vi "Events.vi"(8 "error in (no error)":errorcluster, 11 "LocalEventCollector in":refnum<class "LocalEventCollector.lvclass">) -> (0 "error out":errorcluster, 2 "Events":T1[](array[typedef]), 3 "LocalEventCollector out":refnum<class "LocalEventCollector.lvclass">)   [LabVIEW 2020, in "Vecto.lvlib" / "LocalEventCollector.lvclass"]
uses:
  LocalEventCollector.lvclass
  Event.ctl
  lv-volatus/Volatus/Event Level.ctl
  LocalEventCollector.lvclass/LocalEventCollector.ctl
  lv-volatus/Volatus/Volatus.lvlib
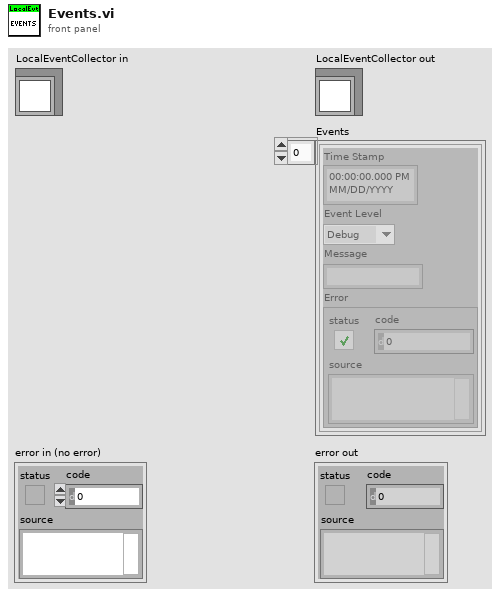
[diagram p1: front panel]
types:
  T1 = typedef "Vecto.lvlib/LocalEventCollector.lvclass/Event.ctl" = cluster{"Time Stamp":timestamp, "Event Level":T2, "Message":string, "Error":errorcluster}
  T2 = typedef "Volatus.lvlib/Event Level.ctl" = enum16{"Debug", "Info", "Warning", "Error"}
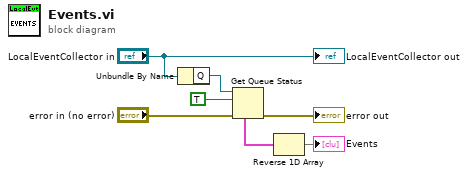
[diagram p0: block diagram]
diagram:
  n1 = Unbundle By Name("LocalEventCollector in") -> ("Q"=w6:refnum<queue>)
  n2 = Get Queue Status(queue=w6, return elements? (F)=TRUE, error in (no error)="error in (no error)") -> (error out=→"error out":errorcluster, elements=w4:T1[])  [unwired: 6 out]
  n3 = Reverse 1D Array(array=w4) -> (reversed array=→"Events":T1[])
  "LocalEventCollector out" <- "LocalEventCollector in"
